vi "Unsubscribe.vi"(8 "error in (no error)":errorcluster, 10 "SubscriptionPolicy":T1, 11 "IMediator In":refnum<class "IMediator.lvclass">) -> (0 "error out":errorcluster, 3 "IMediator Out":refnum<class "IMediator.lvclass">)   [LabVIEW 2020, in "IMediator.lvlib" / "IMediator.lvclass"]
doc: "抽象方法\n取消订阅"
uses:
  IMediator.lvclass
  ISubscriptionPolicy/ISubscriptionPolicy Reference.ctl
  ISubscriptionPolicy/ISubscriptionPolicy.lvclass
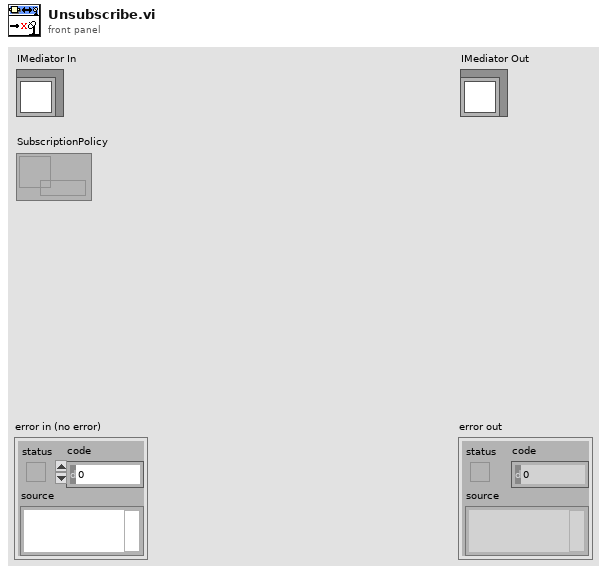
[diagram p1: front panel]
types:
  T1 = typedef "IMediator.lvlib/ISubscriptionPolicy.lvclass/ISubscriptionPolicy Reference.ctl" = refnum<data-value>
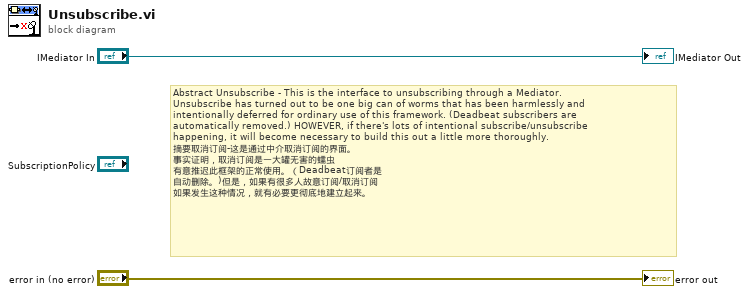
[diagram p0: block diagram]
diagram:
  # "Abstract Unsubscribe - This is the interface to unsubscribing through a Mediator.\nUnsubscribe has turned out to be one big can of worms that has been harmlessly and\nintentionally deferred for ordinary use of this framework. (Deadbeat subscribers are\nautomatically removed.) HOWEVER, if there's lots of intentional subscribe/unsubscribe\nhappening, it will become necessary to build this out a little more thoroughly.\n摘要取消订阅-这是通过中介取消订阅的界面。\n事实证明，取消订阅是一大罐无害的蠕虫\n有意推迟此框架的正常使用。（Deadbeat订阅者是\n自动删除。)但是，如果有很多人故意订阅/取消订阅\n如果发生这种情况，就有必要更彻底地建立起来。"
  "error out" <- "error in (no error)"
  "IMediator Out" <- "IMediator In"
